vi "Atto DRY Interface is Device Connected.vi"(8 "error in (no error)":errorcluster, 11 "isConnected":i32) -> (0 "error out":errorcluster, 2 "function return":i32, 3 "isConnected out":i32)   [LabVIEW 2016, in "attoDRYLib.lvlib"]
doc: "int32_t __cdecl AttoDRY_Interface_isDeviceConnected(int *isConnected);"
uses:
  <userlib>/attoDRYLib/attoDRYLib.lvlib
  <userlib>/attoDRYLib/attoDRYLib.dll
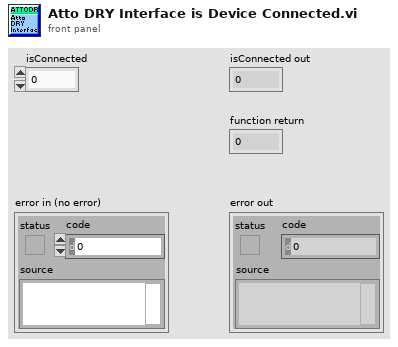
[diagram p1: front panel]
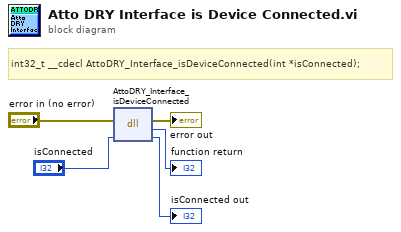
[diagram p0: block diagram]
diagram:
  # "int32_t __cdecl AttoDRY_Interface_isDeviceConnected(int *isConnected);"
  n1 = dll-call lib="C:/Program Files (x86)/National Instruments/LabVIEW 2016/user.lib/attoDRYLib/attoDRYLib.*" fn="AttoDRY_Interface_isDeviceConnected"(error in="error in (no error)", "isConnected"="isConnected") -> (error out=→"error out":errorcluster, →"function return":i32, "isConnected"=→"isConnected out":i32)  [unwired: 2 in, 1 out]
